vi "Read UI State.vi"(8 "error in (no error)":errorcluster, 11 "EmbeddedSMO in":refnum<class "SMO.UI.Embedded.lvclass">) -> (0 "error out":errorcluster, 2 "UI State":T1=enum."Embedded", 3 "EmbeddedSMO out":refnum<class "SMO.UI.Embedded.lvclass">)   [LabVIEW 2016, in "SMO.UI.Embedded.lvclass"]
uses:
  SMO.UI.Embedded.lvclass
  Typedefs/UI State.ctl
  SMO.UI.Embedded.lvclass/SMO.UI.Embedded.ctl
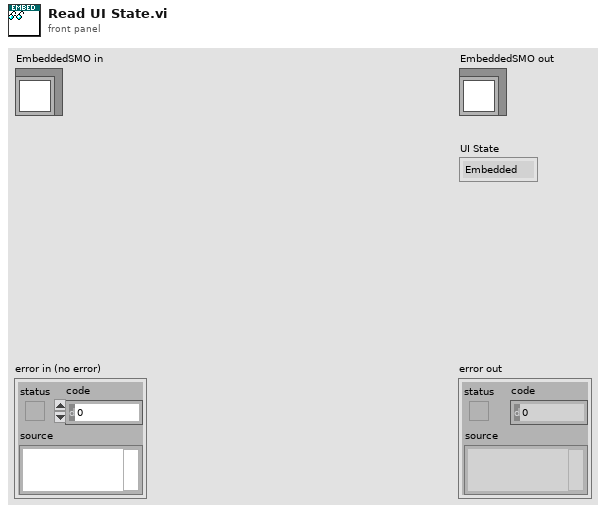
[diagram p1: front panel]
types:
  T1 = typedef "SMO.UI.Embedded.lvclass/UI State.ctl" = enum16{"unknown", "Opened", "Embedded", "Closed"}
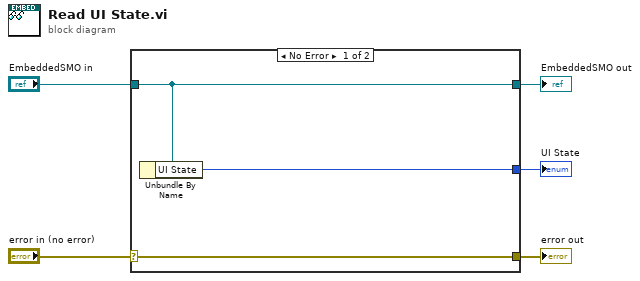
[diagram p0: block diagram]
diagram:
  n1 = case shown="No Error" "error in (no error)" {
    selector: "error in (no error)" -> [w8 w9]
    tunnel: [w8 w9] -> w4
    tunnel: [w7 w10] -> w2
    tunnel: "EmbeddedSMO in" -> [w7 w10]
    tunnel: [w6 _] -> w1
    frame No Error {
      n2 = Unbundle By Name(w7) -> ("UI State"=w6:T1)
    }
    frame Error {
    }
  }
  "error out" <- w4
  "EmbeddedSMO out" <- w2
  "UI State" <- w1
